vi "laser_on_off.vi"() -> ()   [LabVIEW 2017]
panel:
  in  "Slide":u8(slide)=25 min=1 max=100 step=1 scale=1.0..100.0
  in  "Stop Program":bool
  out "Error String":string
  out "error out":errorcluster
  out "Boolean 2":bool
  in  "Boolean":bool
  in  "Identifier":string="LJM_idANY"
  in  "ConnectionType":string="LJM_ctANY"
  in  "DeviceType":string="LJM_dtANY"
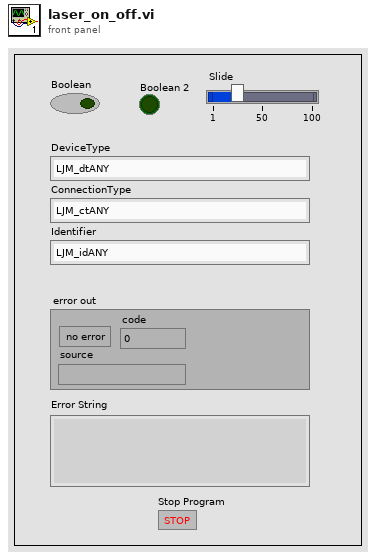
[diagram p1: front panel]
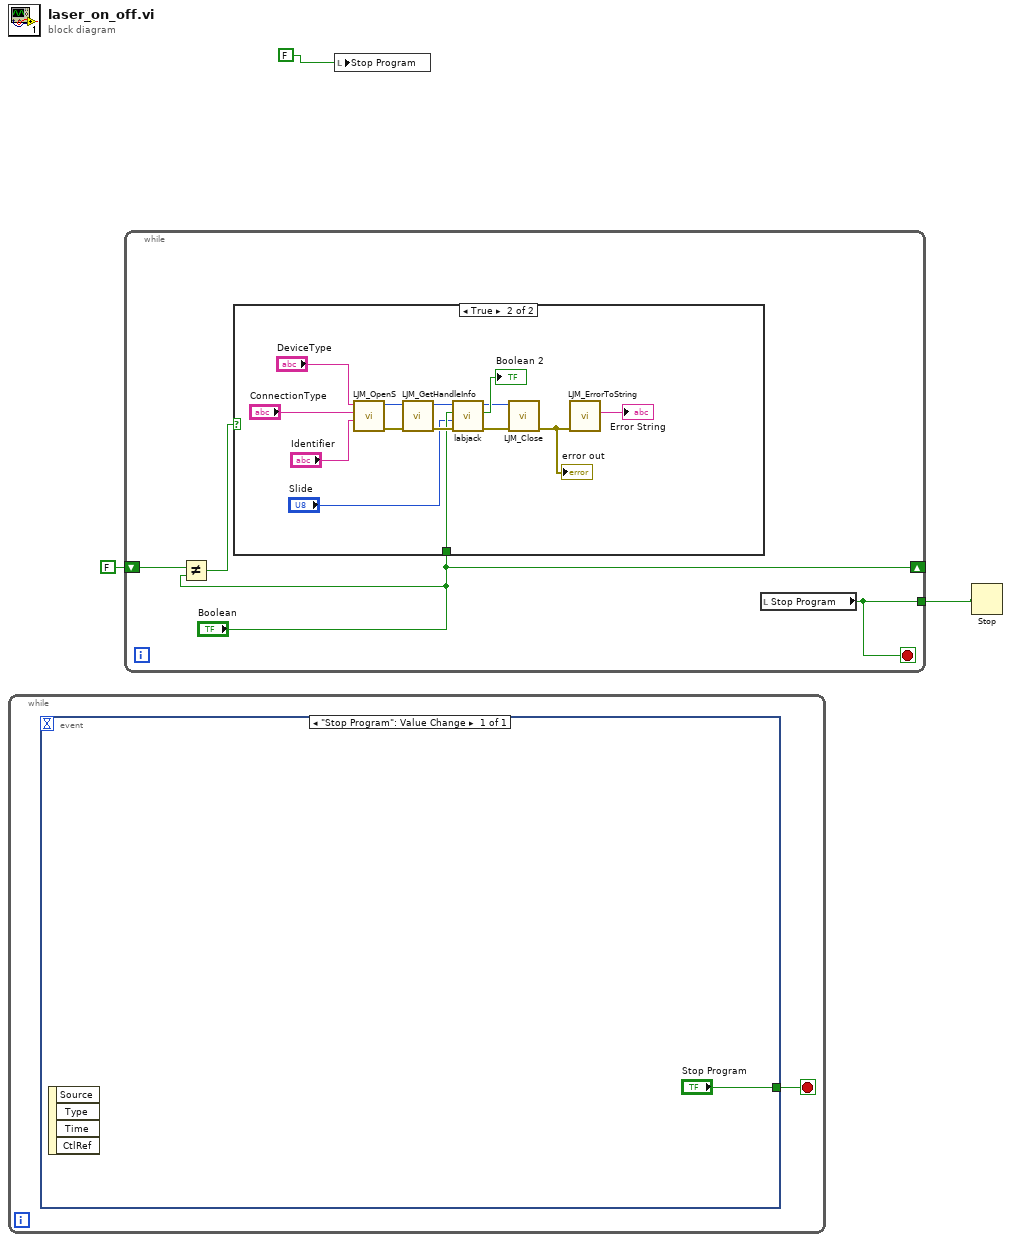
[diagram p0: block diagram]
diagram:
  n1 = while {
    stop <- w4 stop-if-true
    n2 = event shown="[0] \"Stop Program\": Value Change" {
      selector: _ -> [_]
      dyn-events: _ -> [_]
      timeout: _ -> [_]
      tunnel: ["Stop Program"] -> w4
      event "Stop Program": Value Change {
        n3 = event-data() -> ()  [unwired: 1 in, 4 out]
      }
    }
  }
  n4 = while {
    tunnel: [w9] -> w3
    shift-right: ["Boolean"] -> _
    shift-left: FALSE ("Boolean") -> [w8]
    stop <- w9 stop-if-true
    n5 = Not Equal?(x=w8, y="Boolean") -> (x != y?=w6:bool)
    n6 = case shown="True" w6 {
      tunnel: "Boolean" -> [_ w11]
      frame False {
      }
      frame True {
        n7 = call "LJM_OpenS.vi"("Identifier"="Identifier", "ConnectionType"="ConnectionType", "DeviceType"="DeviceType") -> ("error out"=w19:errorcluster, "Handle"=w20:i32)  [unwired: 7 in]
        n8 = call "LJM_GetHandleInfo.vi"("error in"=w19, "Handle In"=w20) -> ("error out"=w17:errorcluster, "Handle Out"=w18:i32)  [unwired: 2 in, 6 out]
        n9 = call "labjack.vi"("error out"=w17, "PwmDtc"="Slide", "Boolean"=w11, "Handle Out"=w18) -> ("error out 2"=w13:errorcluster, "Boolean 2"=→"Boolean 2":bool, "Handle Out 2"=w12:i32)  [unwired: 5 in]
        n10 = call "LJM_Close.vi"("error in"=w13, "Handle"=w12) -> ("error out"=w14:errorcluster)  [unwired: 9 in]
        "error out" <- w14
        n11 = call "LJM_ErrorToString.vi"("error in"=w14) -> ("String"=→"Error String":string)  [unwired: 10 in]
      }
    }
    n12 = local read "Stop Program"() -> (w9:bool)
  }
  n13 = local write "Stop Program"(FALSE) -> ()
  n14 = Stop(stop? (T)=w3) -> ()
